vi "subHideArray.vi"(0 "Array":refnum<vi>[](array[refnum]), 1 "Show":bool) -> ()   [LabVIEW 2020]
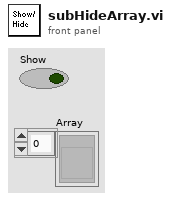
[diagram p1: front panel]
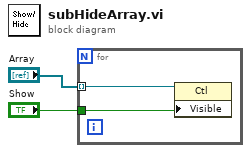
[diagram p0: block diagram]
diagram:
  n1 = for {
    tunnel: "Array" -> [w4] mode=indexing
    tunnel: "Show" -> [w3]
    n2 = property class="Ctl"(reference=w4, "Visible"=w3) -> ()  [unwired: 1 in, 2 out]
  }
